vi "Zaber resolution ---constant.vi"(9 "Montura":T1, 11 "Action":enum16{"Get", "Set"}(ring)) -> (3 "Resolución":dbl[unit])   [LabVIEW 2020]
uses:
  H:/Mi unidad/Departamento de Ingenieria/Investigadores/Gabriel Ramos/Proyecto Monturas v13/LV Source/Type Definitions/Tipos de montura.ctl
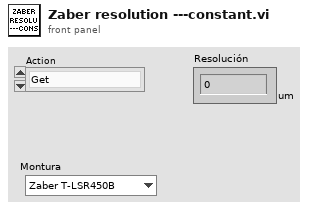
[diagram p1: front panel]
types:
  T1 = typedef "Tipos de montura.ctl" = enum16{"Zaber T-LSR450B", "Zaber-T-LSR300B", "Zaber-T-LSRxxx", "Motor Bipolar", "Motor Unipolar"}
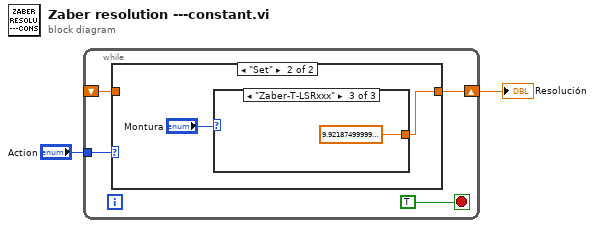
[diagram p0: block diagram]
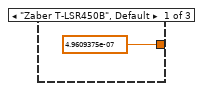
[diagram p3: hidden frame]
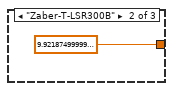
[diagram p4: hidden frame]
diagram:
  n1 = while {
    tunnel: "Action" -> [w4]
    shift-right: [w6] -> w2
    shift-left: _ -> [w3]
    stop <- TRUE stop-if-true
    n2 = case shown="\"Set\"" w4 {
      tunnel: [w7 w8] -> w6
      tunnel: w3 -> [w7 _]
      frame "Get", Default {
      }
      frame "Set" {
        n3 = case shown="\"Zaber-T-LSRxxx\"" "Montura" {
          tunnel: [dbl[unit] 4.9609375e-07 ("Resolución") dbl[unit] 9.921874999999999e-08 ("Resolución") dbl[unit] 9.921874999999999e-08 ("Resolución")] -> w8
          frame "Zaber T-LSR450B", Default {
          }
          frame "Zaber-T-LSR300B" {
          }
          frame "Zaber-T-LSRxxx" {
          }
        }
      }
    }
  }
  "Resolución" <- w2
